vi "Auto_Play_Read_Commands.vi"(10 "Play Name":string) -> (0 "Parameter 4":string[](array[string]), 1 "Parameter 3":string[](array[string]), 2 "Parameter 2":string[](array[string]), 3 "Parameter 1":string[](array[string]), 4 "Concurrent?":string[](array[string]), 5 "Command Names":string[](array[string]))   [LabVIEW 2020]
panel:
  out "List of Commands":string[](array[string])
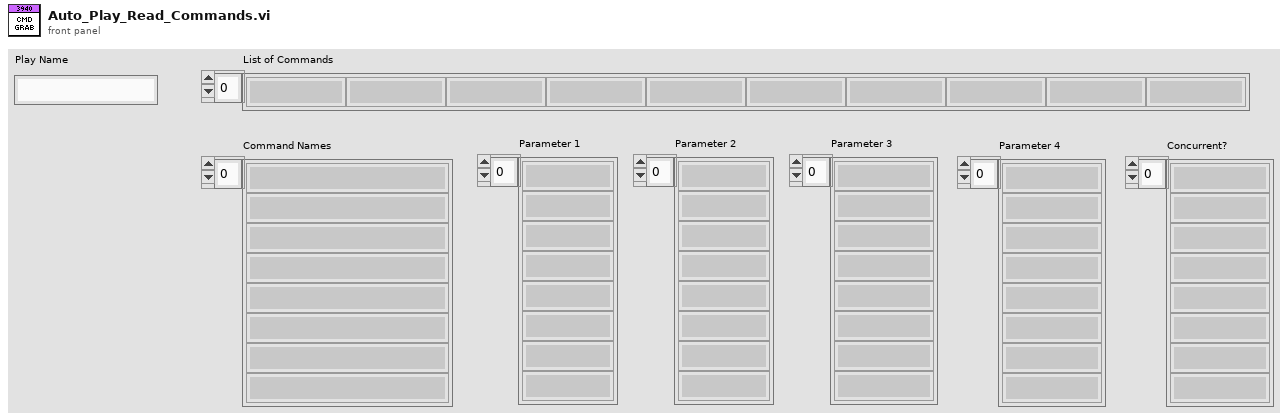
[diagram p1: front panel]
types:
  T1 = enum16{"open", "replace", "create", "open or create", "replace or create", "replace or create with confirmation"}
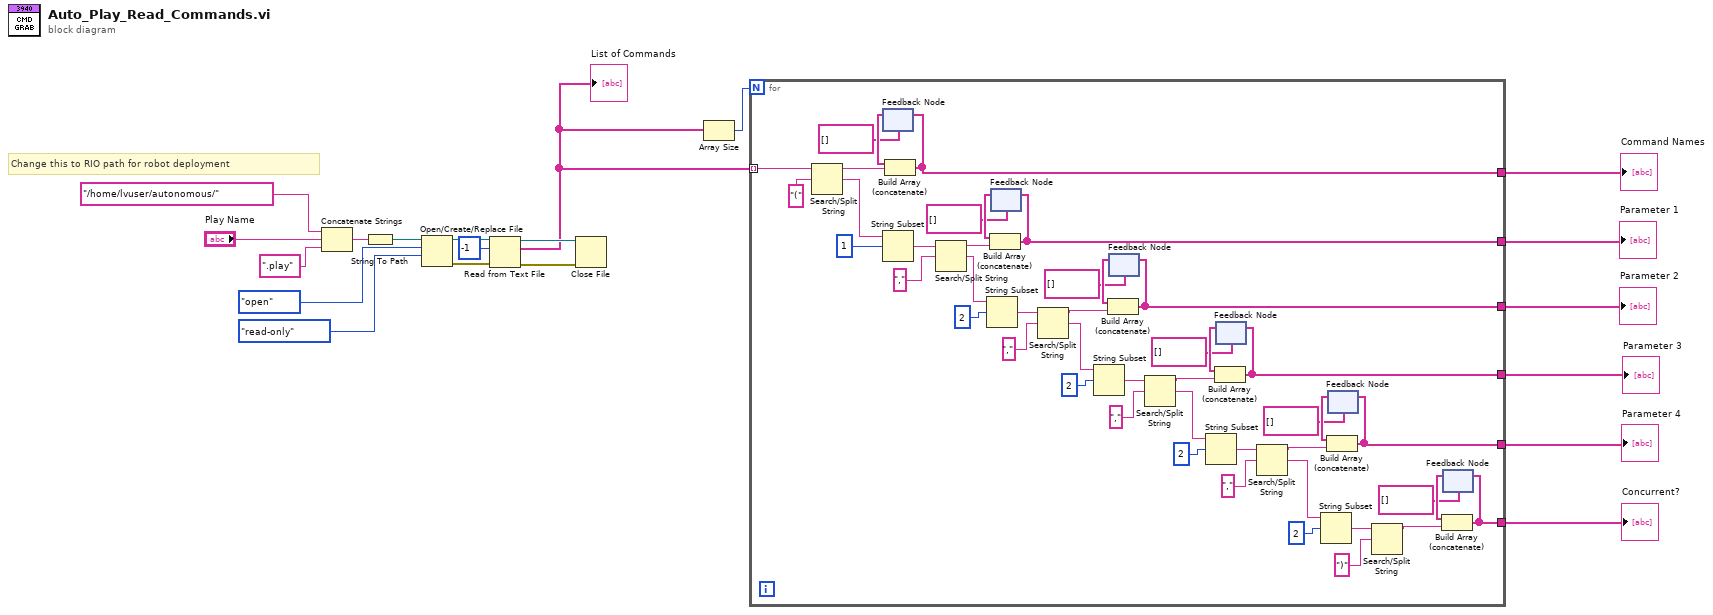
[diagram p0: block diagram]
diagram:
  # "Change this to RIO path for robot deployment"
  n1 = Concatenate Strings("/home/lvuser/autonomous/", "Play Name", ".play") -> (w17:string)
  n2 = String To Path(string=w17) -> (path=w16:path)
  n3 = Open/Create/Replace File(file path (use dialog)=w16, operation (0:open)=T1."open", access (0:read/write)=enum16{"read/write", "read-only", "write-only"}."read-only") -> (refnum out=w12:refnum<file>, error out=w13:errorcluster)  [unwired: 3 in, 1 out]
  n4 = Read from Text File(file (use dialog)=w12, count=-1, error in=w13) -> (refnum out=w10:refnum<file>, text=w7:string[], error out=w9:errorcluster)  [unwired: 1 in, 1 out]
  "List of Commands" <- w7
  n5 = Close File(refnum=w10, error in=w9) -> ()  [unwired: 2 out]
  n6 = Array Size(array=w7) -> (size(s)=w8:i32)
  n7 = for {
    N: w8 -> [_]
    tunnel: w7 -> [w66] mode=indexing
    tunnel: [w64] -> w6
    tunnel: [w53] -> w5
    tunnel: [w45] -> w4
    tunnel: [w37] -> w3
    tunnel: [w29] -> w2
    tunnel: [w21] -> w1
    n8 = Search/Split String(string=w66, search string/char (-)="(") -> (substring before match=w63:string, match + rest of string=w61:string)  [unwired: 1 in, 1 out]
    n9 = feedback #1(string[] []) -> (w62:string[])
    n10 = String Subset(string=w61, offset (0)=1) -> (substring=w59:string)  [unwired: 1 in]
    n11 = Build Array (concatenate)(w62, w63) -> (w64:string[])
    n12 = feedback-in #1(w64) -> ()
    n13 = Search/Split String(string=w59, search string/char (-)=",") -> (substring before match=w57:string, match + rest of string=w52:string)  [unwired: 1 in, 1 out]
    n14 = String Subset(string=w52, offset (0)=2) -> (substring=w50:string)  [unwired: 1 in]
    n15 = feedback #2(string[] []) -> (w55:string[])
    n16 = Build Array (concatenate)(w55, w57) -> (w53:string[])
    n17 = feedback-in #2(w53) -> ()
    n18 = Search/Split String(string=w50, search string/char (-)=",") -> (substring before match=w46:string, match + rest of string=w38:string)  [unwired: 1 in, 1 out]
    n19 = String Subset(string=w38, offset (0)=2) -> (substring=w43:string)  [unwired: 1 in]
    n20 = feedback #3(string[] []) -> (w48:string[])
    n21 = Build Array (concatenate)(w48, w46) -> (w45:string[])
    n22 = feedback-in #3(w45) -> ()
    n23 = Search/Split String(string=w43, search string/char (-)=",") -> (substring before match=w39:string, match + rest of string=w30:string)  [unwired: 1 in, 1 out]
    n24 = String Subset(string=w30, offset (0)=2) -> (substring=w35:string)  [unwired: 1 in]
    n25 = feedback #4(string[] []) -> (w41:string[])
    n26 = Build Array (concatenate)(w41, w39) -> (w37:string[])
    n27 = feedback-in #4(w37) -> ()
    n28 = Search/Split String(string=w35, search string/char (-)=",") -> (substring before match=w31:string, match + rest of string=w22:string)  [unwired: 1 in, 1 out]
    n29 = String Subset(string=w22, offset (0)=2) -> (substring=w27:string)  [unwired: 1 in]
    n30 = feedback #5(string[] []) -> (w33:string[])
    n31 = Build Array (concatenate)(w33, w31) -> (w29:string[])
    n32 = feedback-in #5(w29) -> ()
    n33 = Search/Split String(string=w27, search string/char (-)=")") -> (substring before match=w23:string)  [unwired: 1 in, 2 out]
    n34 = feedback #6(string[] []) -> (w25:string[])
    n35 = Build Array (concatenate)(w25, w23) -> (w21:string[])
    n36 = feedback-in #6(w21) -> ()
  }
  "Command Names" <- w6
  "Parameter 1" <- w5
  "Parameter 2" <- w4
  "Parameter 3" <- w3
  "Parameter 4" <- w2
  "Concurrent?" <- w1
